vi "Calculate_number_of_steps.vi"(11 "Rotation angle [°]":dbl) -> (0 "Number of steps":i32, 3 "Number of steps":string)   [LabVIEW 2021]
doc: "This VI enables to calculate number of Stepper Motor (SM) steps, according to rotation angle for SM step resolution 1/64.\n\nInputs:\n\n(1) Rotation angle [°] - the rotation angle in [°]\n\nOutput:\n(1) Number of steps - the number of the SM steps"
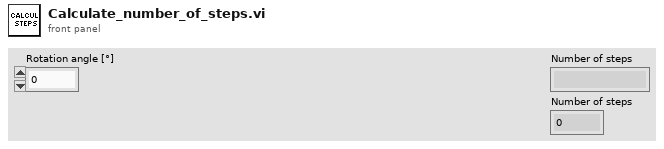
[diagram p1: front panel]
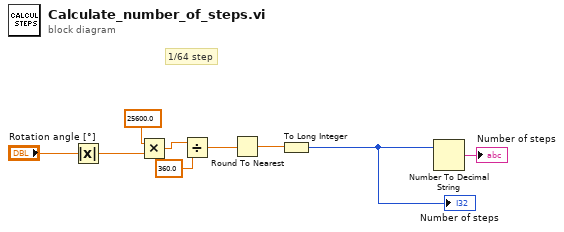
[diagram p0: block diagram]
diagram:
  # "1/64 step"
  n1 = Absolute Value(x="Rotation angle [°]") -> (abs(x)=w5:dbl)
  n2 = Multiply(x=25600.0, y=w5) -> (x*y=w8:dbl)
  n3 = Divide(x=w8, y=360.0) -> (x/y=w2:dbl)
  n4 = Round To Nearest(number=w2) -> (nearest integer value=w1:dbl)
  n5 = To Long Integer(number=w1) -> (32bit integer=w3:i32)
  "Number of steps" <- w3
  n6 = Number To Decimal String(number=w3) -> (decimal integer string=→"Number of steps":string)  [unwired: 1 in]
